vi "IsStartFound.vi"(8 "error in (no error)":errorcluster, 10 "data in":string, 11 "TCP_Client in":refnum<class "TCP_Client.lvclass">) -> (0 "error out":errorcluster, 2 "StartOfMessage":bool, 3 "TCP_Client out":refnum<class "TCP_Client.lvclass">)   [LabVIEW 2023, in "TCP_Client.lvlib" / "TCP_Client.lvclass"]
uses:
  TCP_Client.lvclass
  TCP_Client.lvclass/TCP_Client.ctl
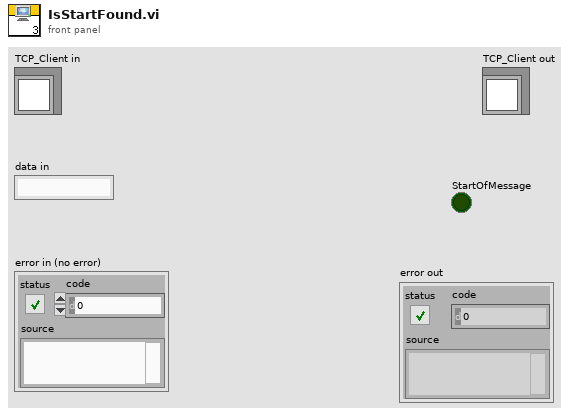
[diagram p1: front panel]
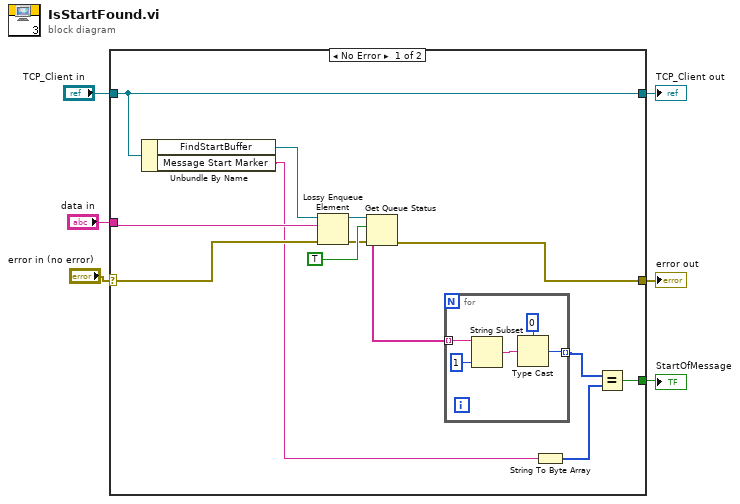
[diagram p0: block diagram]
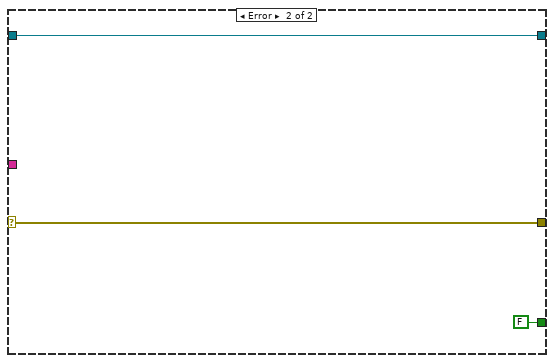
[diagram p2: hidden frame]
diagram:
  n1 = case shown="No Error" "error in (no error)" {
    selector: "error in (no error)" -> [w16 w26]
    tunnel: "TCP_Client in" -> [w8 w27]
    tunnel: "data in" -> [w14 _]
    tunnel: [w9 FALSE] -> w3
    tunnel: [w8 w27] -> w2
    tunnel: [w7 w26] -> w1
    frame No Error {
      n2 = Unbundle By Name(w8) -> ("FindStartBuffer"=w15:refnum<queue>, "Message Start Marker"=w12:string)
      n3 = Lossy Enqueue Element(queue=w15, element=w14, error in (no error)=w16) -> (queue out=w17:refnum<queue>, error out=w18:errorcluster)  [unwired: 2 out]
      n4 = Get Queue Status(queue=w17, return elements? (F)=TRUE, error in (no error)=w18) -> (error out=w7:errorcluster, elements=w13:string[])  [unwired: 6 out]
      n5 = for {
        tunnel: w13 -> [w24] mode=indexing
        tunnel: [w20] -> w11 mode=indexing
        n6 = String Subset(string=w24, length (rest)=1 ("length (rest)")) -> (substring=w22:string)  [unwired: 1 in]
        n7 = Type Cast(type=u8 0, x=w22) -> (*(type *) &x=w20:u8)
      }
      n8 = String To Byte Array(string=w12) -> (unsigned byte array=w10:u8[])
      n9 = Equal?(x=w11, y=w10) -> (x = y?=w9:bool)
    }
    frame Error {
    }
  }
  "error out" <- w1
  "TCP_Client out" <- w2
  "StartOfMessage" <- w3
